vi "FPGA User Variables Host.vi"() -> ()   [LabVIEW 2025]
uses:
  FPGA IP/Types/PWM.Measure.Digital.Result.ctl
  FPGA IP/Types/PWM.Generate.Digital.Convert.Settings.ctl
  FPGA IP/Types/PWM.Measure.Digital.Measurement.ctl
  <vilib>/FPGAPlugInAG/cRIO-9045/niLvFpga_Open_cRIO-9045.vi
  <vilib>/rvi/interface/common/dynamic/niFpgaDynamicAddResources.vi
  <vilib>/FPGAPlugInAG/Dynamic/niLvFpga_Close_Dynamic.vi
  <vilib>/rvi/interface/nirviOpenFPGA/nirviOpenFPGA.xnode
  FPGA Bitfiles/scanengineexampl_FPGATarget_ExampleFPGA_9nPm7+spJUY.lvbitx
  <vilib>/rvi/interface/nirviCloseFPGA/nirviCloseFPGA.xnode
  FPGA IP/Speciality FPGA IO.lvlib
panel:
  in  "PWM Generation Settings":T1={"ACTIVE EDGE"=TRUE, "FREQ"=5.0, "DC"=48.0}
  out "PWM Result":T2
  in  "stop acq":bool
  out "error out":errorcluster
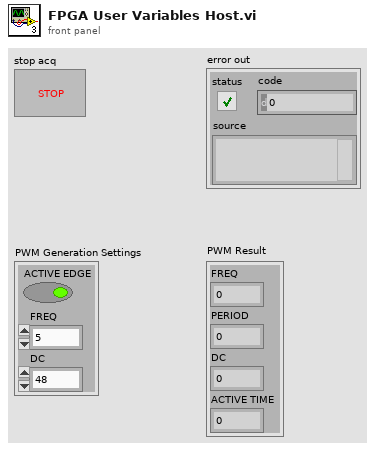
[diagram p1: front panel]
types:
  T1 = typedef "Speciality FPGA IO.lvlib/PWM.Generate.Digital.Convert.Settings.ctl" = cluster{"ACTIVE EDGE":bool, "FREQ":sgl, "DC":sgl}
  T2 = typedef "Speciality FPGA IO.lvlib/PWM.Measure.Digital.Result.ctl" = cluster{"FREQ":sgl, "PERIOD":sgl, "DC":sgl, "ACTIVE TIME":sgl}
  T3 = typedef "Speciality FPGA IO.lvlib/PWM.Measure.Digital.Measurement.ctl" = cluster{"ACTIVE TICKS":u32, "INACTIVE TICKS":u32, "ACQ TICKS":u32}
  T4 = typedef "Speciality FPGA IO.lvlib/PWM.Generate.Digital.Settings.ctl" = cluster{"ACTIVE EDGE":bool, "ACTIVE TICKS":u32, "INACTIVE TICKS":u32}
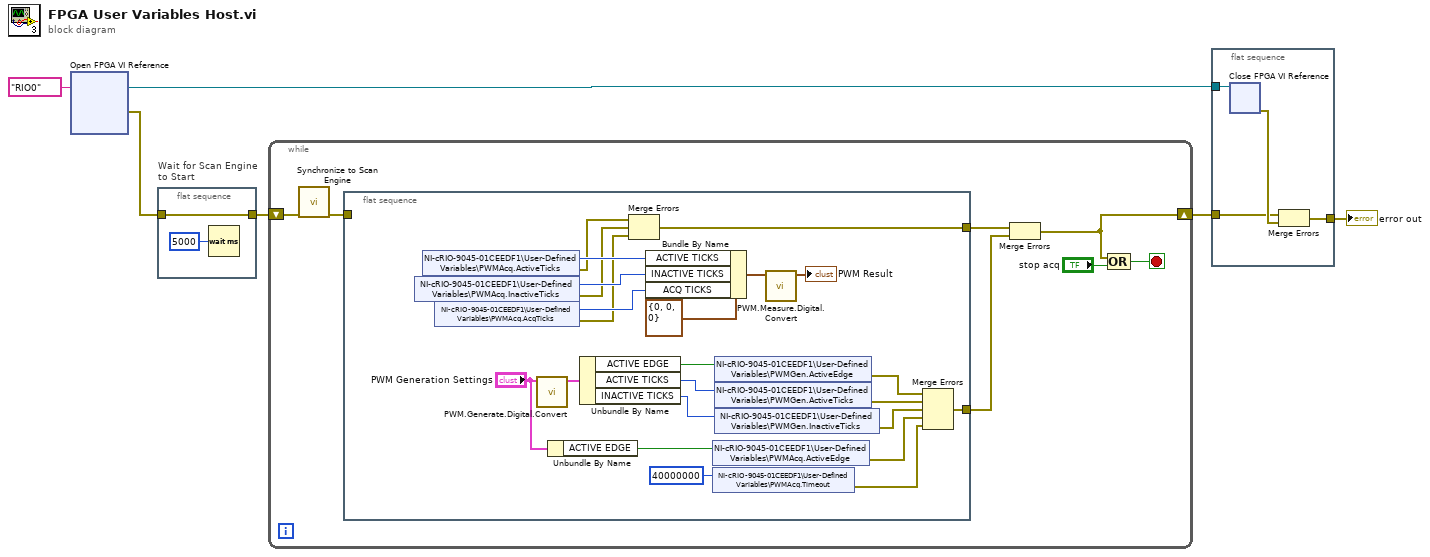
[diagram p0: block diagram]
diagram:
  n1 = xnode "Open FPGA VI Reference"("resource name"=tag "RIO0") -> ("FPGA VI Reference Out"=w5:refnum<k20>, "error out"=w3:errorcluster)  [unwired: 1 in]
  n2 = flat-sequence "Wait for Scan Engine\nto Start" {
    tunnel: [w8] -> w2
    tunnel: w3 -> [w8]
    frame #0 {
      n3 = Wait (ms)(milliseconds to wait=u32 5000) -> ()  [unwired: 1 out]
    }
  }
  n4 = while {
    shift-right: [w9] -> w1
    shift-left: w2 -> [w15]
    stop <- w13 stop-if-true
    n5 = call <vilib>:"Synchronize to Scan Engine.vi"("error in (no error)"=w15) -> ("error out"=w12:errorcluster)  [unwired: 9 in, 1 out]
    n6 = flat-sequence {
      tunnel: w12 -> [_]
      tunnel: [w17] -> w11
      tunnel: [w16] -> w10
      frame #0 {
        n7 = shared-variable "NI-cRIO-9045-01CEEDF1\\User-Defined Variables\\PWMAcq.InactiveTicks"() -> (w36:u32, error out=w24:errorcluster)  [unwired: 1 in]
        n8 = shared-variable "NI-cRIO-9045-01CEEDF1\\User-Defined Variables\\PWMAcq.ActiveTicks"() -> (w35:u32, error out=w25:errorcluster)  [unwired: 1 in]
        n9 = shared-variable "NI-cRIO-9045-01CEEDF1\\User-Defined Variables\\PWMAcq.AcqTicks"() -> (w37:u32, error out=w23:errorcluster)  [unwired: 1 in]
        n10 = call "PWM.Generate.Digital.Convert.vi"("Settings"="PWM Generation Settings") -> ("Settings"=w30:T4)  [unwired: 10 in]
        n11 = Unbundle By Name("PWM Generation Settings") -> ("ACTIVE EDGE"=w26:bool)
        n12 = Unbundle By Name(w30) -> ("ACTIVE EDGE"=w31:bool, "ACTIVE TICKS"=w32:u32, "INACTIVE TICKS"=w33:u32)
        n13 = Merge Errors(w25, w24, w23) -> (w17:errorcluster)
        n14 = Bundle By Name(cluster=T3 {"ACTIVE TICKS"=0, "INACTIVE TICKS"=0, "ACQ TICKS"=0} ("Measurement"), "ACTIVE TICKS"=w35, "INACTIVE TICKS"=w36, "ACQ TICKS"=w37) -> (w34:T3)
        n15 = shared-variable "NI-cRIO-9045-01CEEDF1\\User-Defined Variables\\PWMAcq.ActiveEdge"(w26) -> (error out=w19:errorcluster)  [unwired: 1 in]
        n16 = shared-variable "NI-cRIO-9045-01CEEDF1\\User-Defined Variables\\PWMAcq.Timeout"(u32 40000000 ("PWMAcq.Timeout")) -> (error out=w18:errorcluster)  [unwired: 1 in]
        n17 = shared-variable "NI-cRIO-9045-01CEEDF1\\User-Defined Variables\\PWMGen.ActiveEdge"(w31) -> (error out=w22:errorcluster)  [unwired: 1 in]
        n18 = shared-variable "NI-cRIO-9045-01CEEDF1\\User-Defined Variables\\PWMGen.ActiveTicks"(w32) -> (error out=w21:errorcluster)  [unwired: 1 in]
        n19 = shared-variable "NI-cRIO-9045-01CEEDF1\\User-Defined Variables\\PWMGen.InactiveTicks"(w33) -> (error out=w20:errorcluster)  [unwired: 1 in]
        n20 = call "PWM.Measure.Digital.Convert.vi"("Measurement"=w34) -> ("Result"=→"PWM Result":T2)  [unwired: 10 in]
        n21 = Merge Errors(w22, w21, w20, w19, w18) -> (w16:errorcluster)
      }
    }
    n22 = Merge Errors(w11, w10) -> (w9:errorcluster)
    n23 = Compound Arithmetic op=OR(w9, "stop acq") -> (w13:bool)
  }
  n24 = flat-sequence {
    tunnel: w5 -> [w42]
    tunnel: w1 -> [w40]
    tunnel: [w39] -> w4
    frame #0 {
      n25 = xnode "Close FPGA VI Reference"("FPGA VI Reference In"=w42) -> ("error out"=w41:errorcluster)  [unwired: 1 in]
      n26 = Merge Errors(w40, w41) -> (w39:errorcluster)
    }
  }
  "error out" <- w4
